vi "GUI Update Trigger Mode Selector.vi"(1 "capabilities":T1, 2 "trig mode ref":refnum<vi>) -> (0 "has parameters?":bool)   [LabVIEW 2018]
doc: "Updates trigger menu based on the capabilities of the selected HW."
uses:
  adc/ADC Trig Mode Source.ctl
  adc/ADC Capabilities.ctl
  adc/ADC Sampling Rate Step Mode.ctl
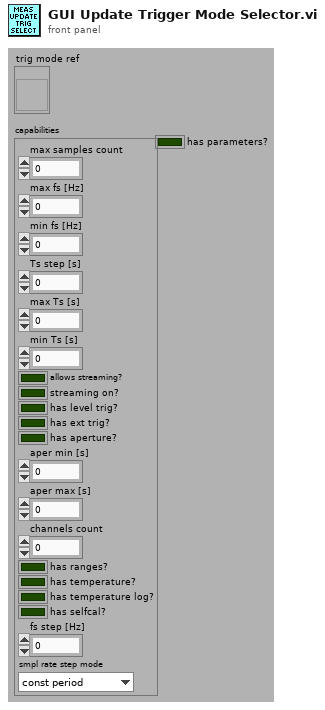
[diagram p1: front panel]
types:
  T1 = typedef "ADC Capabilities.ctl" = cluster{"max samples count":i64, "max fs [Hz]":ext, "min fs [Hz]":ext, "Ts step [s]":ext, "max Ts [s]":ext, "min Ts [s]":ext, "allows streaming?":bool, "streaming on?":bool, "has level trig?":bool, "has ext trig?":bool, "has aperture?":bool, "aper min [s]":dbl, "aper max [s]":dbl, "channels count":i32, "has ranges?":bool, "has temperature?":bool, "has temperature log?":bool, "has selfcal?":bool, "fs step [Hz]":ext, "smpl rate step mode":T2}
  T2 = typedef "ADC Sampling Rate Step Mode.ctl" = enum16{"const period", "const frequency"}
  T3 = typedef "ADC Trig Mode Source.ctl" = enum16{"Immediate", "External", "Level"}
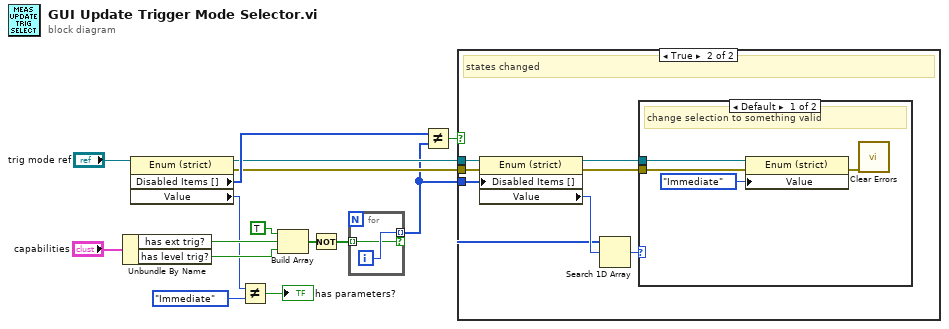
[diagram p0: block diagram]
diagram:
  n1 = Unbundle By Name("capabilities") -> ("has ext trig?"=w7:bool, "has level trig?"=w6:bool)
  n2 = property class="Enum (strict)"(reference="trig mode ref") -> (reference out=w9:refnum<vi>, error out=w10:errorcluster, "Disabled Items []"=w11:i32[], "Value"=w5:T3)  [unwired: 1 in]
  n3 = Not Equal?(x=w5, y=ADC_Trig_Mode_Source."Immediate") -> (x != y?=→"has parameters?":bool)
  n4 = Build Array(TRUE, w7, w6) -> (w13:bool[])
  n5 = Not(x=w13) -> (.not. x?=w2:bool[])
  n6 = for {
    tunnel: w2 -> [w16] mode=indexing
    tunnel: [w17] -> w1 mode=indexing if=w16
    i -> [w17]
  }
  n7 = Not Equal?(x=w11, y=w1) -> (x != y?=w8:bool)
  n8 = case shown="True" w8 {
    tunnel: w1 -> [_ w20]
    tunnel: w10 -> [_ w19]
    tunnel: w9 -> [_ w18]
    frame False {
      # "states unchaged"
    }
    frame True {
      # "states changed"
      n9 = property class="Enum (strict)"(reference=w18, error in=w19, "Disabled Items []"=w20) -> (reference out=w22:refnum<vi>, error out=w21:errorcluster, "Value"=w24:T3)
      n10 = Search 1D Array(1D array=w20, element=w24) -> (index of element=w23:i32)  [unwired: 1 in]
      n11 = case shown="Default" w23 {
        tunnel: w22 -> [w28 _]
        tunnel: w21 -> [w27 _]
        frame Default {
          # "change selection to something valid"
          n12 = property class="Enum (strict)"(reference=w28, error in=w27, "Value"=ADC_Trig_Mode_Source."Immediate") -> (error out=w25:errorcluster)  [unwired: 1 out]
          n13 = call <vilib>:"Clear Errors.vi"("error in (no error)"=w25) -> ()  [unwired: 5 in, 2 out]
        }
        frame -1 {
        }
      }
    }
  }
